vi "Day 3 (Part One).vi"() -> ()   [LabVIEW 2021]
panel:
  out "sum":i32
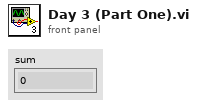
[diagram p1: front panel]
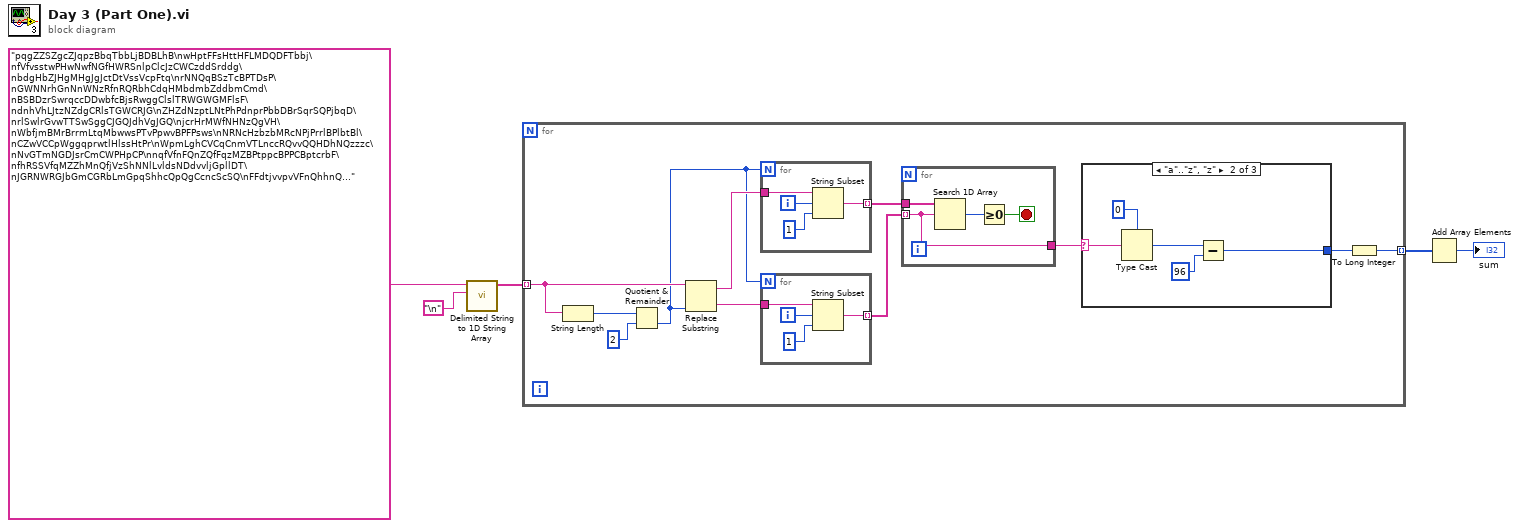
[diagram p0: block diagram]
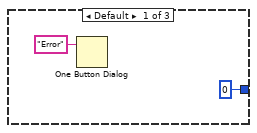
[diagram p2: hidden frame]
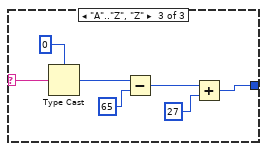
[diagram p3: hidden frame]
diagram:
  n1 = call <vilib>:"Delimited String to 1D String Array.vi"("delimiter"="\n", "delimited string"="pqgZZSZgcZJqpzBbqTbbLjBDBLhB\nwHptFFsHttHFLMDQDFTbbj\nfVfvsstwPHwNwfNGfHWRSnlpClcJzCWCzddSrddg\nbdgHbZJHgMHgJgJctDtVssVcpFtq\nrNNQqBSzTcBPTDsP\nGWNNrhGnNnWNzRfnRQRbhCdqHMbdmbZddbmCmd\nBSBDzrSwrqccDDwbfcBjsRwggClslTRWGWGMFlsF\ndnhVhLJtzNZdgCRlsTGWCRJG\nZHZdNzptLNtPhPdnprPbbDBrSqrSQPjbqD\nrlSwlrGvwTTSwSggCJGQJdhVgJGQ\njcrHrMWfNHNzQgVH\nWbfjmBMrBrrmLtqMbwwsPTvPpwvBPFPsws\nNRNcHzbzbMRcNPjPrrlBPlbtBl\nCZwVCCpWggqprwtlHlssHtPr\nWpmLghCVCqCnmVTLnccRQvvQQHDhNQzzzc\nNvGTmNGDJsrCmCWPHpCP\nnqfVfnFQnZQfFqzMZBPtppcBPPCBptcrbF\nfhRSSVfqMZZhMnQfjVzShNNlLvldsNDdvvljGpllDT\nJGRNWRGJbGmCGRbLmGpqShhcQpQgCcncScSQ\nFFdtjvvpvVFnQhhnQ...") -> ("string array"=w3:string[])  [unwired: 9 in]
  n2 = for {
    tunnel: w3 -> [w14] mode=indexing
    tunnel: [w6] -> w2 mode=indexing
    n3 = String Length(string=w14) -> (length=w16:i32)
    n4 = Quotient & Remainder(x=w16, y=2) -> (floor(x/y)=w9:i32)  [unwired: 1 out]
    n5 = Replace Substring(2:w9, 5:w14) -> (0:w13:string, 1:w12:string)  [unwired: 2 in]
    n6 = for {
      N: w9 -> [_]
      tunnel: w12 -> [w24]
      tunnel: [w21] -> w11 mode=indexing
      i -> [w22]
      n7 = String Subset(string=w24, offset (0)=w22, length (rest)=1 ("length (rest)")) -> (substring=w21:string)
    }
    n8 = for {
      N: w9 -> [_]
      tunnel: w13 -> [w28]
      tunnel: [w25] -> w10 mode=indexing
      i -> [w26]
      n9 = String Subset(string=w28, offset (0)=w26, length (rest)=1 ("length (rest)")) -> (substring=w25:string)
    }
    n10 = for {
      tunnel: w10 -> [w17] mode=indexing
      tunnel: w11 -> [w20]
      tunnel: [w17] -> w7
      stop <- w18 stop-if-true
      n11 = Search 1D Array(1D array=w20, element=w17) -> (index of element=w19:i32)  [unwired: 1 in]
      n12 = Greater Or Equal To 0?(x=w19) -> (x >= 0?=w18:bool)
    }
    n13 = case shown="\"a\"..\"z\", \"z\"" w7 {
      selector: w7 -> [_ w31 w39]
      tunnel: [u8 0 w33 w36] -> w8
      frame Default {
        n14 = One Button Dialog(message="Error") -> ()  [unwired: 1 in, 1 out]
      }
      frame "a".."z", "z" {
        n15 = Type Cast(type=u8 0, x=w31) -> (*(type *) &x=w32:u8)
        n16 = Subtract(x=w32, y=u8 96) -> (x-y=w33:u8)
      }
      frame "A".."Z", "Z" {
        n17 = Type Cast(type=u8 0, x=w39) -> (*(type *) &x=w40:u8)
        n18 = Subtract(x=w40, y=u8 65) -> (x-y=w38:u8)
        n19 = Add(x=w38, y=u8 27) -> (x+y=w36:u8)
      }
    }
    n20 = To Long Integer(number=w8) -> (32bit integer=w6:i32)
  }
  n21 = Add Array Elements(numeric array=w2) -> (sum=→"sum":i32)
